vi "saveSequenceFile.vi"(9 "fileName":string, 10 "NewSequenceFile":refnum<k7>, 11 "Sequence Context In":refnum<k7>) -> (0 "error out":errorcluster)   [LabVIEW 2011]
doc: "Saves the sequence file to the current sequence file directory with the specified name."
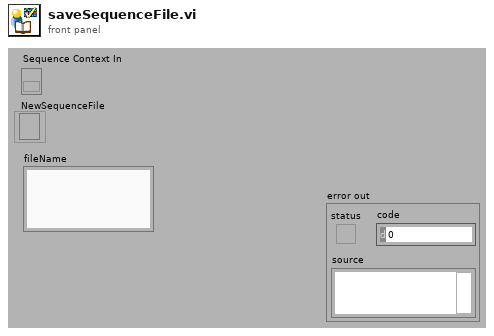
[diagram p1: front panel]
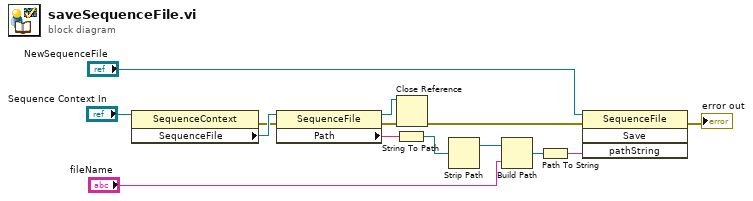
[diagram p0: block diagram]
diagram:
  n1 = property class="SequenceContext"(reference="Sequence Context In") -> (error out=w5:errorcluster, "SequenceFile"=w12:refnum<k7>)  [unwired: 1 in, 1 out]
  n2 = property class="SequenceFile"(reference=w12, error in=w5) -> (reference out=w3:refnum<k7>, error out=w4:errorcluster, "Path"=w11:string)
  n3 = String To Path(string=w11) -> (path=w10:path)
  n4 = Close Reference(reference=w3, error in (no error)=w4) -> (error out=w2:errorcluster)
  n5 = Strip Path(path=w10) -> (stripped path=w9:path)  [unwired: 1 out]
  n6 = Build Path(base path=w9, name or relative path="fileName") -> (appended path=w7:path)
  n7 = Path To String(path=w7) -> (string=w6:string)
  n8 = invoke class="SequenceFile" method="Save"(reference="NewSequenceFile", error in=w2, "pathString"=w6) -> (error out=→"error out":errorcluster)  [unwired: 1 in, 3 out]
